vi "Configure Service Request.vi"(8 "error in (no error)":errorcluster {"code" format="%.0x"}, 9 "Reason (StbMAV)":i32(ring)=1 items=["StbMAV"=1, "Stb Error Queue"=2, "EsrOPC"=4, "Esr Query Error"=8, "Esr Device Error"=16, "Esr Execution Error"=32, "Esr Command Error"=64, "Esr User Request"=128, "Ques Voltage"=256, "Ques Current"=512, "Ques Time"=1024, "Ques Power"=2048, "Ques Temperature"=4096, "Ques Frequency"=8192, "Ques Phase"=16384, "Ques Modulation"=32768, "Ques Calibration"=65536, "Ques Instrument"=131072], 11 "instrument handle":refnum<k15>) -> (0 "error out":errorcluster {"code" format="%.0x"}, 3 "instrument handle out":refnum<k15>)   [LabVIEW 2009, in "Keysight XSAn.lvlib"]
doc: "Clears all the enable registers. It then sets the appropriate transition filters and enable registers so when the specified event(s) occur(s) the instrument requests service. All other events are disabled from generating a service request. To detect a service request the client application must poll the status byte using the Status.SerialPoll method or Status.Register property and test the request service bit.\n\nSupported Models: All supported"
uses:
  <instrlib>/Keysight XSAn/Keysight XSAn.lvlib
  AgXSAn.dll
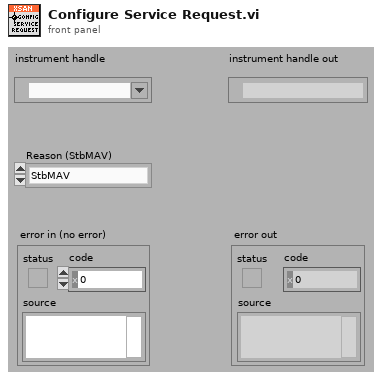
[diagram p1: front panel]
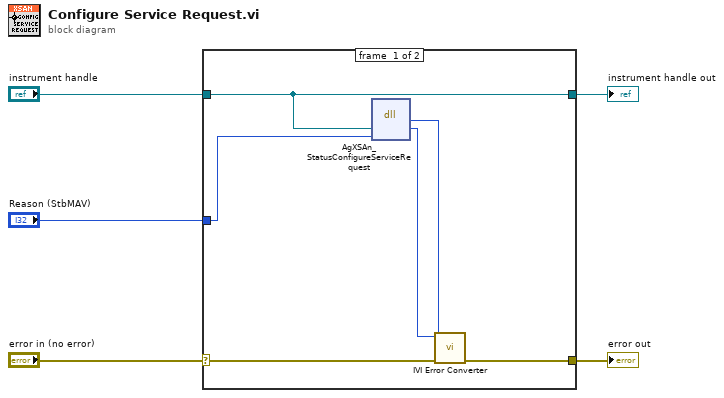
[diagram p0: block diagram]
diagram:
  n1 = case shown="No Error" "error in (no error)" {
    selector: "error in (no error)" -> [w9 w13]
    tunnel: [w8 w13] -> w5
    tunnel: "instrument handle" -> [w6 w12]
    tunnel: "Reason (StbMAV)" -> [w7 _]
    tunnel: [w6 w12] -> w1
    frame #0 {
      n2 = dll-call lib="AgXSAn**.dll" fn="AgXSAn_StatusConfigureServiceRequest"("Vi"=w6, "Reason"=w7) -> (w10:i32, "Vi"=w11:u32)  [unwired: 4 in, 2 out]
      n3 = call <instrlib>:"IVI Error Converter.vi"("error in (no error)"=w9, "IVI error code (0)"=w10, "instrument handle"=w11) -> ("error out"=w8:errorcluster)  [unwired: 7 in, 1 out]
    }
    frame #1 {
    }
  }
  "error out" <- w5
  "instrument handle out" <- w1
